vi "Modbust PM5100 Read.vi"() -> ()   [LabVIEW 2022 SP3]
uses:
  <vilib>/NI Modbus.llb/MB Serial Master Query Read Holding Registers (poly).vi
panel:
  out "C-N":dbl
  out "B-N":dbl
  out "A-N":dbl
  out "Input Registers":u16[](array[numeric])
  in  "stop":bool
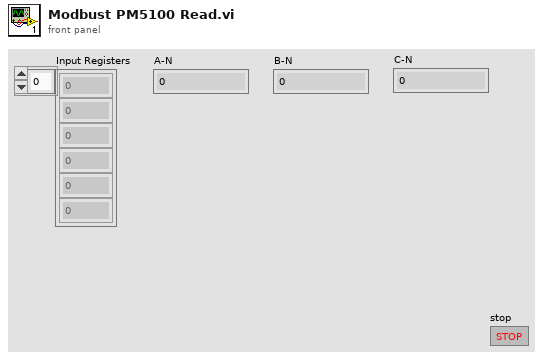
[diagram p1: front panel]
types:
  T1 = cluster{"Mode":enum16{"RTU", "ASCII"}, "Slave Address":u8}
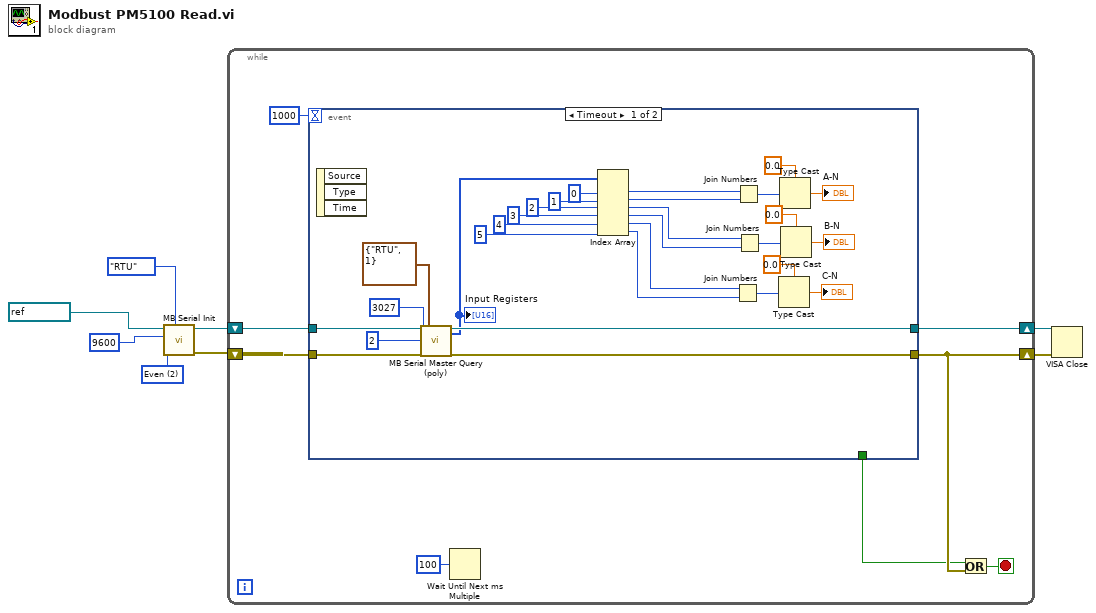
[diagram p0: block diagram]
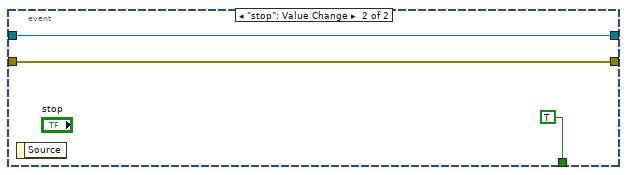
[diagram p2: hidden frame]
diagram:
  w4 = u16 2 items=["None", "Odd", "Even", "Mark", "Space"] ("Parity")
  n1 = call <vilib>:"MB Serial Init.vi"("Mode"=enum16{"RTU", "ASCII"}."RTU", "Parity"=w4, "Baud Rate"=u32 9600, "VISA resource name"=refnum<visa-resource-name> "COM7") -> ("error out"=w7:errorcluster, "VISA resource name out"=w8:refnum<visa-resource-name>)  [unwired: 6 in]
  n2 = while {
    shift-right: [w14] -> w2
    shift-left: w8 -> [w16]
    shift-right: [w11] -> w1
    shift-left: w7 -> [w15]
    stop <- w12 stop-if-true
    n3 = event shown="[0] Timeout" {
      selector: _ -> [_ _]
      dyn-events: _ -> [_ _]
      timeout: 1000 -> [_ _]
      tunnel: w16 -> [w45 w46]
      tunnel: w15 -> [w44 w47]
      tunnel: [w40 w46] -> w14
      tunnel: [w17 w47] -> w11
      tunnel: [_ TRUE] -> w9
      event Timeout {
        n4 = event-data() -> ()  [unwired: 1 in, 3 out]
        n5 = call-poly <vilib>:"MB Serial Master Query (poly).vi"("VISA resource name"=w45, "Starting Address"=u16 3027, "Quantity"=u16 2, "error in"=w44, "Serial Parameters"=T1 {"Mode"=enum."RTU", "Slave Address"=1}) -> ("VISA resource name out"=w40:refnum<visa-resource-name>, "Holding Registers"=w39:u16[], "error out"=w17:errorcluster)  [unwired: 11 in, 1 out]
        "Input Registers" <- w39
        n6 = Index Array(array=w39, index #1=0 ("index"), index #2=1 ("index"), index #3=2 ("index"), index #4=3 ("index"), index #5=4 ("index"), index #6=5 ("index")) -> (element #1=w33:u16, element #2=w32:u16, element #3=w24:u16, element #4=w23:u16, element #5=w21:u16, element #6=w20:u16)
        n7 = Join Numbers(hi=w21, lo=w20) -> ((hi.lo)=w22:u32)
        n8 = Join Numbers(hi=w33, lo=w32) -> ((hi.lo)=w36:u32)
        n9 = Join Numbers(hi=w24, lo=w23) -> ((hi.lo)=w27:u32)
        n10 = Type Cast(type=sgl 0.0, x=w22) -> (*(type *) &x=→"C-N":sgl)
        n11 = Type Cast(type=sgl 0.0, x=w36) -> (*(type *) &x=→"A-N":sgl)
        n12 = Type Cast(type=sgl 0.0, x=w27) -> (*(type *) &x=→"B-N":sgl)
      }
      event "stop": Value Change {
        n13 = event-data() -> ()  [unwired: 1 in, 1 out]
      }
    }
    n14 = Wait Until Next ms Multiple(millisecond multiple=u32 100) -> ()  [unwired: 1 out]
    n15 = Or(x=w9, y=w11) -> (x .or. y?=w12:bool)
  }
  n16 = VISA Close(VISA resource name=w2, error in (no error)=w1) -> ()  [unwired: 1 out]
